vi "RT Driver VI.vi"(7 "Operation":T1, 11 "Device Reference in":T2 format="%.0x") -> (0 "Error Code":i32)   [LabVIEW 2023, in "Embedded TDMS Logger Engine.lvlib"]
uses:
  Embedded TDMS Logger Engine.lvlib
  <vilib>/NI VeriStand/Custom Device API/Custom Device Item Ref.ctl
  <vilib>/NI VeriStand/Custom Device API/Hardware Interface Driver VI Operation.ctl
  Shared/Compiled.Settings.ctl
  Shared/FileData.ctl
  Shared/GroupData.ctl
  Shared/Meta Data Item.ctl
  Shared/ChannelData.ctl
  <vilib>/NI VeriStand/Custom Device API/Data Reference.ctl
  Shared/SegmentOptions.ctl
  <vilib>/NI/NIVS Inline Async API/_VS Inline Async API/VS Inline Async API/VS Inline Async API.lvclass
  <vilib>/NI/NIVS Inline Async API/_VS Inline Async API/VS Inline Async API/VS Inline Async API.lvclass/VS Inline Async API.ctl
  <vilib>/NI/NIVS Inline Async API/_Data Access Engine/Data Access Engine/Data Access Engine.lvclass/Data Access Engine.ctl
  <vilib>/NI/NIVS Inline Async API/_Data Access Engine/Access Type Classes/Write/Write.lvclass/Write.ctl
  <vilib>/NI/NIVS Inline Async API/_Data Access Engine/Access Type Classes/ReadWrite/ReadWrite.lvclass/ReadWrite.ctl
  <vilib>/NI/NIVS Inline Async API/_Data Access Engine/Access Type Classes/Read/Read.lvclass/Read.ctl
  <vilib>/NI/NIVS Inline Async API/_Data Access Engine/Data Access Engine/Methods/Data.Engine.Read Data from HW.vi
  <vilib>/NI/NIVS Inline Async API/_VS Inline Async API/Error Handling Process/SubVIs/Error.GetError.vi
  <vilib>/NI/NIVS Inline Async API/_Data Access Engine/Data Access Engine/Methods/Data.Engine.Write Data to HW.vi
  <vilib>/NI/NIVS Inline Async API/_Data Access Engine/Access Type Classes/ReadWrite/ReadWrite.EngineData.vi
  <vilib>/NI/NIVS Inline Async API/_Data Access Engine/Access Type Classes/Write/Write.EngineData.vi
  <vilib>/NI/NIVS Inline Async API/_Data Access Engine/Access Type Classes/Read/Read.EngineData.vi
  <vilib>/NI VeriStand/Custom Device API/NI VeriStand - Get Channel Value by Data Reference.vi
  <vilib>/NI VeriStand/Custom Device API/NI VeriStand - Set Channel Value by Data Reference.vi
  <vilib>/NI VeriStand/Custom Device API/NI VeriStand - Get Channel Values by Block Data Reference.vi
  Embedded TDMS Logger.Async.vi
  Shared/Constants.vi
  <vilib>/NI VeriStand/Custom Device API/Get Item Property (Variant).vi
  <vilib>/NI VeriStand/Custom Device API/Global Data Refs.vi
  <vilib>/NI VeriStand/Custom Device API/Custom Device API.lvlib
  <vilib>/NI VeriStand/Custom Device Tools/Custom Device Utility Library/Custom Device Utility Library.lvlib
  Shared/Embedded TDMS Logger Shared.lvlib
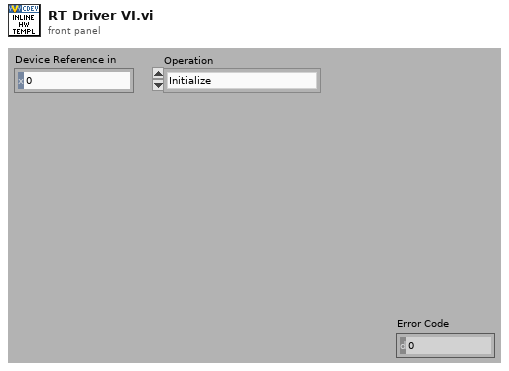
[diagram p1: front panel]
types:
  T1 = typedef "Custom Device API.lvlib/Hardware Interface Driver VI Operation.ctl" = enum16{"Initialize", "Start", "Read Data from HW", "Write Data to HW", "Close"}
  T2 = typedef "Custom Device API.lvlib/Custom Device Item Ref.ctl" = u64
  T3 = typedef "Embedded TDMS Logger Shared.lvlib/Compiled.Settings.ctl" = cluster{"Name":string, "Async Init Timeout":u16, "File Data":T4, "Segment Files":bool, "Segment Every":dbl, "Trigger?":bool, "Segment by":T9, "Trigger Ref":T8}
  T4 = typedef "Embedded TDMS Logger Shared.lvlib/FileData.ctl" = cluster{"Date Captured":string, "Directory":string, "Name":string, "Groups":T5[], "Meta Data":T6[]}
  T5 = typedef "Embedded TDMS Logger Shared.lvlib/GroupData.ctl" = cluster{"Data Rate":string, "Meta Data":T6[], "Channels":T7[], "Name":string}
  T6 = typedef "Embedded TDMS Logger Shared.lvlib/Meta Data Item.ctl" = cluster{"Key":string, "Value":string}
  T7 = typedef "Embedded TDMS Logger Shared.lvlib/ChannelData.ctl" = cluster{"Name":string, "Meta Data":T6[], "Data Reference":T8, "Wfm?":bool, "Increment":dbl}
  T8 = typedef "Custom Device API.lvlib/Data Reference.ctl" = i32
  T9 = typedef "SegmentOptions.ctl" = enum16{"Time (s)", "Size (MB)"}
  T10 = cluster{"Async":refnum<class "VS Inline Async API.lvclass">, "Compiled.Settings":T3}
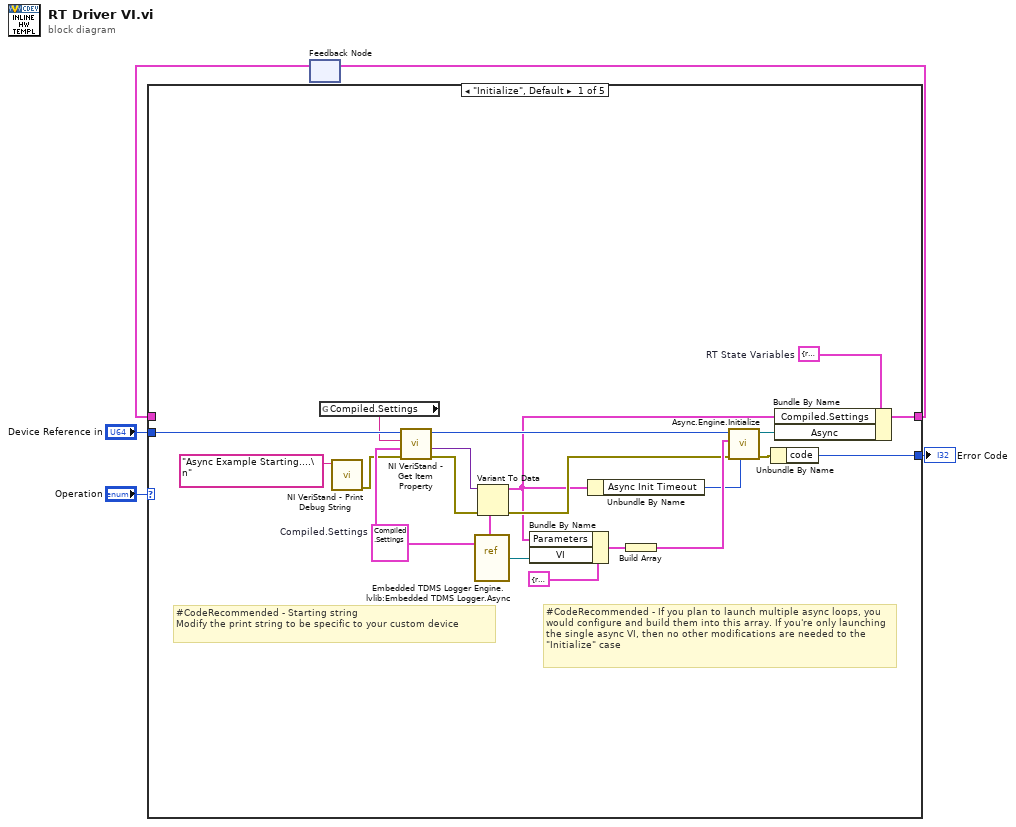
[diagram p0: block diagram]
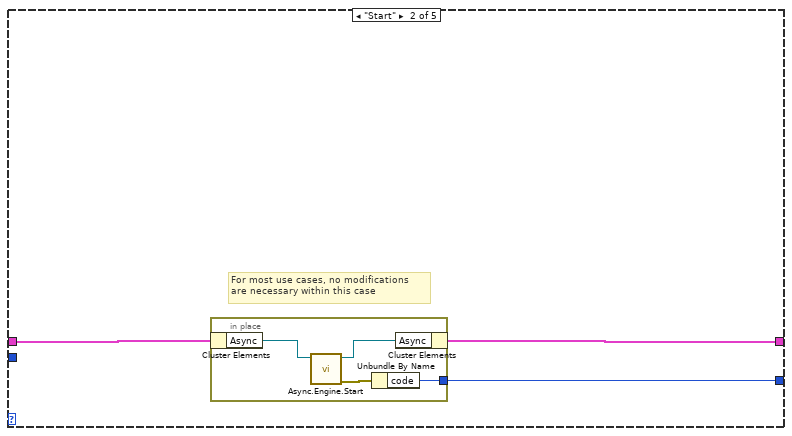
[diagram p2: hidden frame]
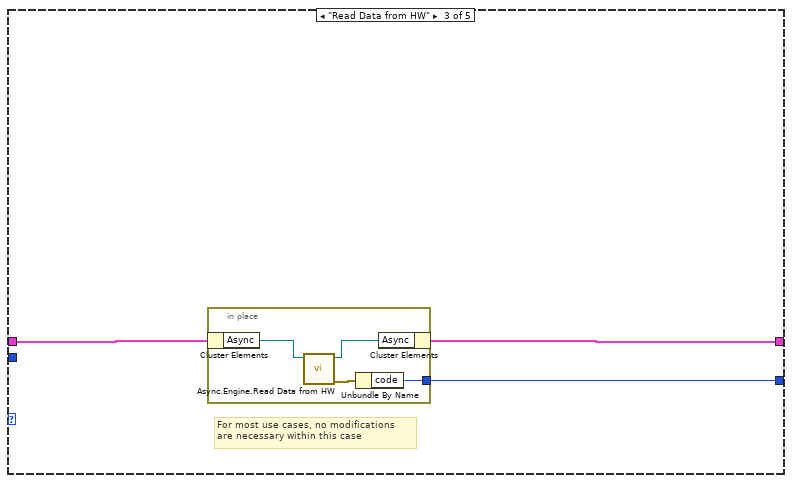
[diagram p3: hidden frame]
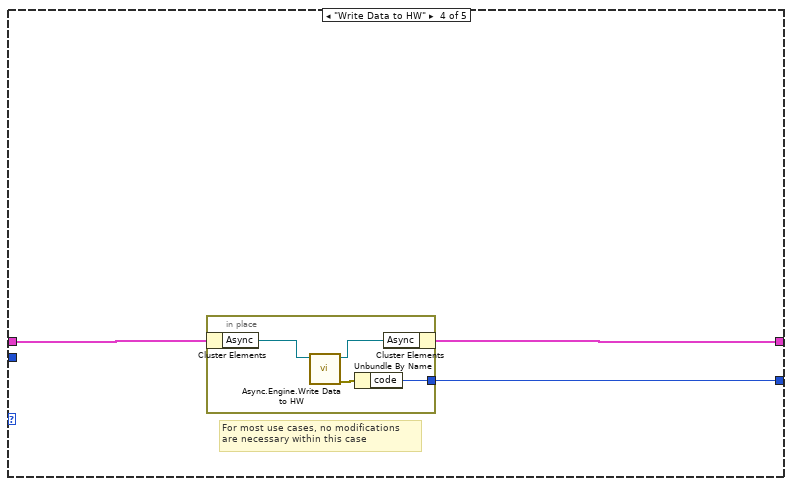
[diagram p4: hidden frame]
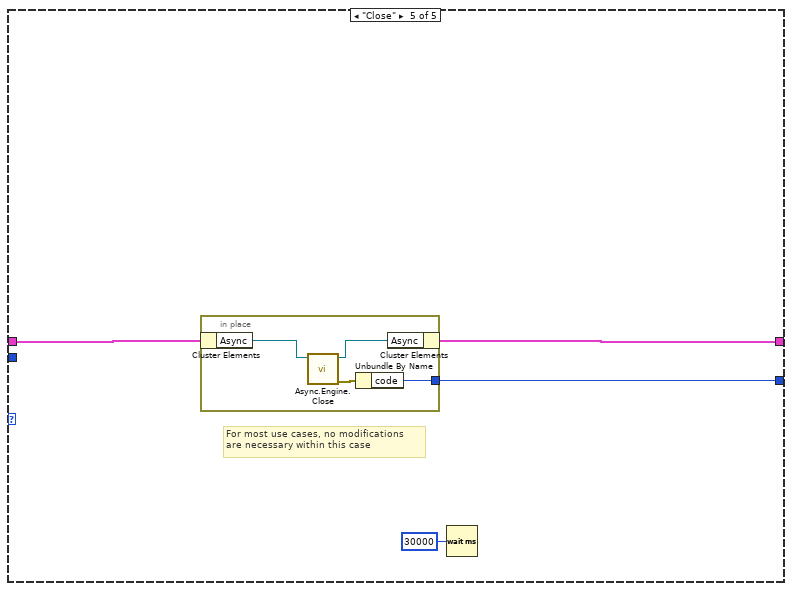
[diagram p5: hidden frame]
diagram:
  n1 = feedback #1() -> (w3:T10)  [unwired: 1 out]
  n2 = case shown="\"Initialize\", Default" "Operation" {
    tunnel: [w23 w28 w33 w40 w49] -> w4
    tunnel: w3 -> [_ w26 w35 w41 w50]
    tunnel: "Device Reference in" -> [w20 _ _ _ _]
    tunnel: [w25 w27 w34 w42 w48] -> w1
    frame "Initialize", Default {
      w14 = T10 {"Async"=refnum, "Compiled.Settings"={"Name"="", "Async Init Timeout"=0, "File Data"={"Date Captured"="", "Directory"="", "Name"="", "Groups"=[], "Meta Data"=[]}, "Segment Files"=FALSE, "Segment Every"=0.0, "Trigger?"=FALSE, "Segment by"=enum."Size (MB)", "Trigger Ref"=0}}  # RT State Variables
      w15 = T3 {"Name"="", "Async Init Timeout"=0, "File Data"={"Date Captured"="", "Directory"="", "Name"="", "Groups"=[], "Meta Data"=[]}, "Segment Files"=FALSE, "Segment Every"=0.0, "Trigger?"=FALSE, "Segment by"=enum."Size (MB)", "Trigger Ref"=0}  # Compiled.Settings
      # "#CodeRecommended - Starting string\nModify the print string to be specific to your custom device"
      # "#CodeRecommended - If you plan to launch multiple async loops, you would configure and build them into this array. If you're only launching the single async VI, then no other modifications are needed to the \"Initialize\" case"
      n3 = global read "Constants.vi" "Compiled.Settings"() -> (w17:string)
      n4 = call <vilib>:"NI VeriStand - Print Debug String.vi"("Message"="Async Example Starting....\n") -> ("error out"=w10:errorcluster)  [unwired: 10 in]
      n5 = call-poly <vilib>:"NI VeriStand - Get Item Property.vi"("error in (no error)"=w10, "Default Value"=w15, "Property Name"=w17, "Item Ref in"=w20) -> ("error out"=w19:errorcluster, "Value"=w18:variant, "Item Ref out"=w11:T2)  [unwired: 4 in, 1 out]
      n6 = vi-ref "Embedded TDMS Logger Engine.lvlib:Embedded TDMS Logger.Async.vi"() -> (w8:refnum<vi>)
      n7 = Variant To Data(error in=w19, type=w15, Variant=w18) -> (data=w7:T3, error out=w12:errorcluster)
      n8 = Bundle By Name(cluster=cluster{"VI":refnum<vi>, "Parameters":variant} {"VI"=refnum, "Parameters"=variant} ("Process"), "Parameters"=w7, "VI"=w8) -> (w21:cluster{"VI":refnum<vi>, "Parameters":variant})
      n9 = Unbundle By Name(w7) -> ("Async Init Timeout"=w6:u16)
      n10 = Build Array(w21) -> (w13:cluster{"VI":refnum<vi>, "Parameters":variant}[])
      n11 = call <vilib>:"Async.Engine.Initialize.vi"("Timeout (ms) (5000)"=w6, "error in (no error)"=w12, "Processes"=w13, "Custom Device Ref"=w11) -> ("error out"=w16:errorcluster, "Async"=w24:refnum<class "VS Inline Async API.lvclass">)  [unwired: 6 in]
      n12 = Unbundle By Name(w16) -> ("code"=w25:i32)
      n13 = Bundle By Name(cluster=w14, "Compiled.Settings"=w7, "Async"=w24) -> (w23:T10)
    }
    frame "Start" {
      # "For most use cases, no modifications \nare necessary within this case"
      n14 = in-place {
        in-place-border: [w29] -> w27
        n15 = in-place-cluster #2(w26) -> ("Async"=w32:refnum<class "VS Inline Async API.lvclass">)
        n16 = call <vilib>:"Async.Engine.Start.vi"("VS Inline Async API in"=w32) -> ("error out"=w30:errorcluster, "VS Inline Async API out"=w31:refnum<class "VS Inline Async API.lvclass">)  [unwired: 9 in]
        n17 = Unbundle By Name(w30) -> ("code"=w29:i32)
        n18 = in-place-cluster #2("Async"=w31) -> (w28:T10)
      }
    }
    frame "Read Data from HW" {
      # "For most use cases, no modifications \nare necessary within this case"
      n19 = in-place {
        in-place-border: [w37] -> w34
        n20 = in-place-cluster #3(w35) -> ("Async"=w39:refnum<class "VS Inline Async API.lvclass">)
        n21 = call <vilib>:"Async.Engine.Read Data from HW.vi"("Async in"=w39) -> ("error out"=w36:errorcluster, "Async out"=w38:refnum<class "VS Inline Async API.lvclass">)  [unwired: 9 in]
        n22 = Unbundle By Name(w36) -> ("code"=w37:i32)
        n23 = in-place-cluster #3("Async"=w38) -> (w33:T10)
      }
    }
    frame "Write Data to HW" {
      # "For most use cases, no modifications \nare necessary within this case"
      n24 = in-place {
        in-place-border: [w46] -> w42
        n25 = in-place-cluster #4(w41) -> ("Async"=w44:refnum<class "VS Inline Async API.lvclass">)
        n26 = call <vilib>:"Async.Engine.Write Data to HW.vi"("VS Inline Async API in"=w44) -> ("error out"=w45:errorcluster, "VS Inline Async API out"=w43:refnum<class "VS Inline Async API.lvclass">)  [unwired: 9 in]
        n27 = Unbundle By Name(w45) -> ("code"=w46:i32)
        n28 = in-place-cluster #4("Async"=w43) -> (w40:T10)
      }
    }
    frame "Close" {
      # "For most use cases, no modifications \nare necessary within this case"
      n29 = in-place {
        in-place-border: [w52] -> w48
        n30 = in-place-cluster #5(w50) -> ("Async"=w54:refnum<class "VS Inline Async API.lvclass">)
        n31 = call <vilib>:"Async.Engine.Close.vi"("Async in"=w54) -> ("error out"=w51:errorcluster, "Async out"=w53:refnum<class "VS Inline Async API.lvclass">)  [unwired: 9 in]
        n32 = Unbundle By Name(w51) -> ("code"=w52:i32)
        n33 = in-place-cluster #5("Async"=w53) -> (w49:T10)
      }
      n34 = Wait (ms)(milliseconds to wait=u32 30000) -> ()  [unwired: 1 out]
    }
  }
  "Error Code" <- w1
  n35 = feedback-in #1(w4) -> ()
